vi "Responsive Mock Call Template VI.vi"(8 "error in (no error)":errorcluster, 11 "Mock In":refnum<class "Responsive Mock.lvclass">) -> (0 "error out":errorcluster, 3 "Mock Out":refnum<class "Responsive Mock.lvclass">)   [LabVIEW 2020, in "Templates.lvlib"]
uses:
  Templates.lvlib
  Framework/Responsive Mock/Responsive Mock.lvclass
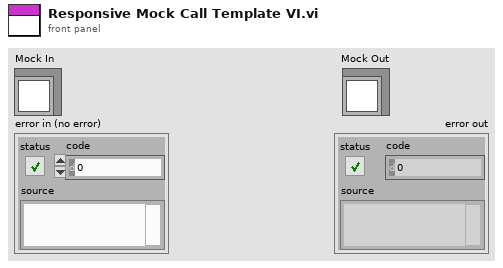
[diagram p1: front panel]
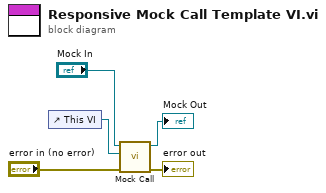
[diagram p0: block diagram]
diagram:
  n1 = control-ref of="This VI"() -> (w5:refnum<vi>)
  n2 = call "Mock Call.vi"("error in (no error)"="error in (no error)", "VI Called"=w5, "Mock In"="Mock In") -> ("error out"=→"error out":errorcluster, "Mock Out"=→"Mock Out":refnum<class "Responsive Mock.lvclass">)  [unwired: 7 in]
